vi "Read Major Frames.vi"(8 "error in":errorcluster, 11 "channel ref in":refnum<k20>) -> (0 "error out":errorcluster, 2 "major frames":T1[](array[typedef]), 3 "channel ref out":refnum<k20>)   [LabVIEW 2020, in "MIL-STD 1553 Import.lvlib"]
uses:
  MIL-STD 1553 Import.lvlib
  Shared/Major Frame Definition.ctl
  3d0c63c2-7e3f-461a-ae28-8bb8601cebbc.vi
  3d0c63c2-7e3f-461a-ae28-8bb8601cebbc.vi/b1e6fcf8-dac1-42d2-b1fe-151afe06dbd4.vi
  Constants.vi
  <vilib>/Utility/error.llb/Error Cluster From Error Code.vi
  <vilib>/xml/NI_XML.lvlib
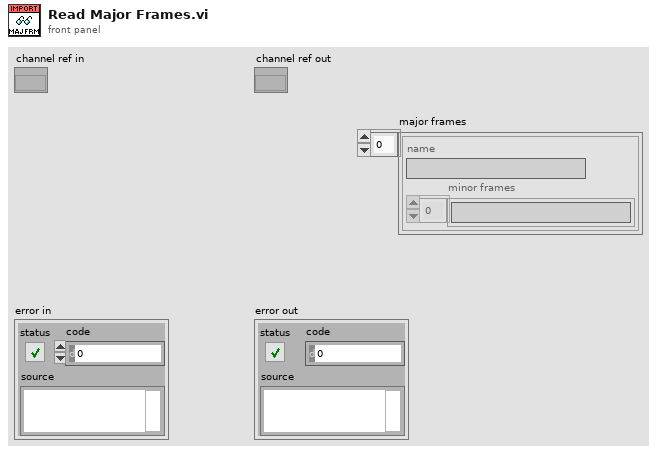
[diagram p1: front panel]
types:
  T1 = typedef "Major Frame Definition.ctl" = cluster{"name":string, "minor frames":string[]}
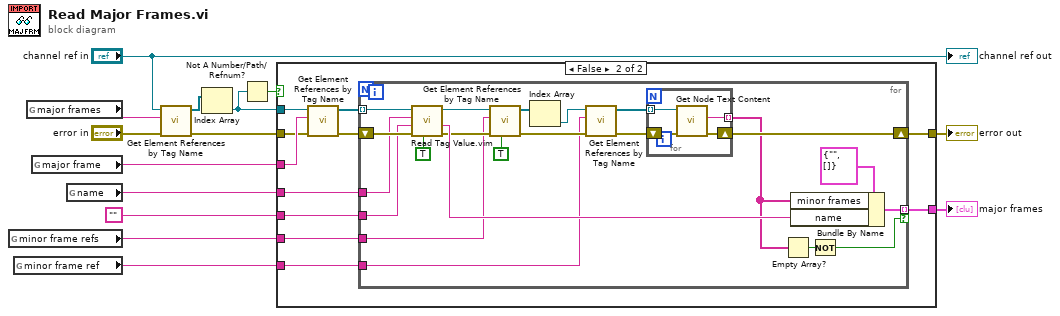
[diagram p0: block diagram]
diagram:
  n1 = global read "Constants.vi" "minor frame refs"() -> (w2:string)
  n2 = global read "Constants.vi" "minor frame ref"() -> (w1:string)
  n3 = global read "Constants.vi" "major frames"() -> (w5:string)
  n4 = global read "Constants.vi" "major frame"() -> (w14:string)
  n5 = global read "Constants.vi" "name"() -> (w12:string)
  n6 = call "Get Element References by Tag Name.vi"("error in"="error in", "tag name"=w5, "node in"="channel ref in") -> ("error out"=w7:errorcluster, "array of elements"=w9:refnum<k20>[])  [unwired: 7 in]
  n7 = Index Array(array=w9) -> (element=w6:refnum<k20>)  [unwired: 1 in]
  n8 = Not A Number/Path/Refnum?(number/path/refnum=w6) -> (NaN/Path/Refnum?=w3:bool)
  n9 = case shown="False" w3 {
    tunnel: w14 -> [_ w26]
    tunnel: [w15 w24] -> w13
    tunnel: w12 -> [_ w22]
    tunnel: "" -> [_ w21]
    tunnel: [_ w20] -> w10
    tunnel: w7 -> [w15 w19]
    tunnel: w6 -> [_ w18]
    tunnel: w2 -> [_ w17]
    tunnel: w1 -> [_ w16]
    frame True {
    }
    frame False {
      n10 = call "Get Element References by Tag Name.vi"("error in"=w19, "tag name"=w26, "node in"=w18) -> ("error out"=w23:errorcluster, "array of elements"=w25:refnum<k20>[])  [unwired: 7 in]
      n11 = for {
        shift-right: [w30] -> w24
        shift-left: w23 -> [w48]
        tunnel: w25 -> [w47] mode=indexing
        tunnel: w22 -> [w46]
        tunnel: w21 -> [w45]
        tunnel: [w42] -> w20 mode=indexing if=w27
        tunnel: w17 -> [w37]
        tunnel: w16 -> [w33]
        n12 = call "Read Tag Value.vim"("required (F)"=TRUE, "error in"=w48, "default"=w45, "tag name"=w46, "node in"=w47) -> ("error out"=w39:errorcluster, "value"=w43:string, "node out"=w40:refnum<k20>)  [unwired: 4 in]
        n13 = call "Get Element References by Tag Name.vi"("required (F)"=TRUE, "error in"=w39, "tag name"=w37, "node in"=w40) -> ("error out"=w34:errorcluster, "array of elements"=w36:refnum<k20>[])  [unwired: 6 in]
        n14 = Index Array(array=w36) -> (element=w35:refnum<k20>)  [unwired: 1 in]
        n15 = call "Get Element References by Tag Name.vi"("error in"=w34, "tag name"=w33, "node in"=w35) -> ("error out"=w31:errorcluster, "array of elements"=w32:refnum<k20>[])  [unwired: 7 in]
        n16 = for {
          tunnel: w32 -> [w52] mode=indexing
          shift-right: [w50] -> w30
          shift-left: w31 -> [w51]
          tunnel: [w49] -> w29 mode=indexing
          n17 = call <vilib>:"Get Node Text Content.vi"("error in (no error)"=w51, "node in"=w52) -> ("error out"=w50:errorcluster, "node text"=w49:string)  [unwired: 7 in, 1 out]
        }
        n18 = Empty Array?(array=w29) -> (empty?=w28:bool)
        n19 = Bundle By Name(cluster=T1 {"name"="", "minor frames"=[]} ("major frame definition"), "minor frames"=w29, "name"=w43) -> (w42:T1)
        n20 = Not(x=w28) -> (.not. x?=w27:bool)
      }
    }
  }
  "error out" <- w13
  "major frames" <- w10
  "channel ref out" <- "channel ref in"
